vi "CubeDrive.vi"   [LabVIEW 2012]
uses:
  State_Machine_Enum.ctl
  <vilib>/Rock Robotics/WPI/RobotDrive/WPI_RobotDriveGetSetRefNum.vi
  Robot Global Data.vi
types:
  T1 = typedef "State_Machine_Enum.ctl" = enum16{"Idle", "Start", "Do", "Stop", "Init"}
  T2 = typedef "WPI_RobotDriveDevRef.ctl" = cluster{"DevStatus":errorcluster, "Motors[]":T3[], "Square Inputs":bool, "Max Output":dbl, "Isochronous":bool}
  T3 = typedef "WPI_MotorControlDeviceRef.ctl" = cluster{"DeviceStatus":errorcluster, "Type":enum16{"PWM", "CAN"}, "PWM":cluster{"Digital Module":T4, "PWM Channel":T5, "DeadBand":T6}, "CAN":cluster{"Device Number":u8, "Control Mode":T7, "Semaphore":T8, "Max Vout":dbl}, "Invert":bool, "TransformRef":T9, "InvTransformRef":T9}
  T4 = typedef "FPGA_TypedefDigitalModule.ctl" = enum16{"Digital Module 1", "Digital Module 2"}
  T5 = typedef "FPGA_DIOPWMChannel.ctl" = enum8{"PWM 1", "PWM 2", "PWM 3", "PWM 4", "PWM 5", "PWM 6", "PWM 7", "PWM 8", "PWM 9", "PWM 10", "Invalid"}
  T6 = typedef "WPI_PWMDeadband.ctl" = cluster{"Name":string, "maxPositivePwm":i32, "minPositivePwm":i32, "centerPwm":i32, "maxNegativePwm":i32, "minNegativePwm":i32, "angularRange":u16}
  T7 = typedef "WPI_CANJaguar_ControlMode.ctl" = enum8{"Percent VBus", "Current", "Speed", "Position", "Voltage"}
  T8 = typedef "Semaphore RefNum" = refnum<k1>
  T9 = typedef "WPI_PWMTransform_ConPane.ctl" = refnum<vi>
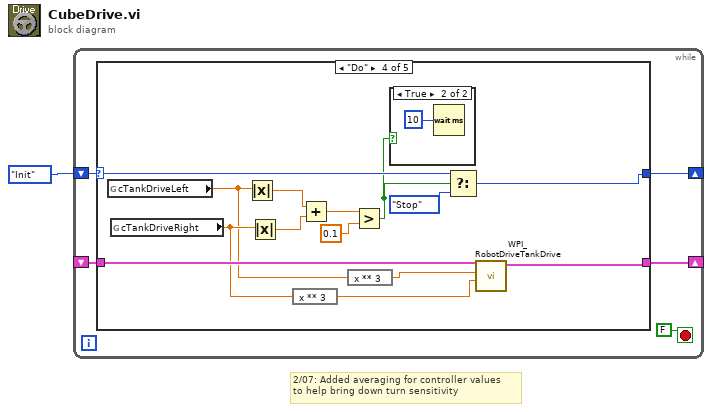
[diagram p0: block diagram]
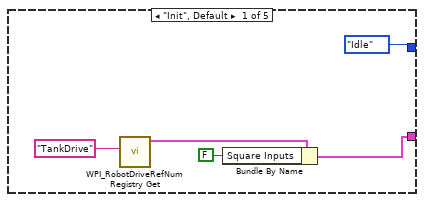
[diagram p2: hidden frame]
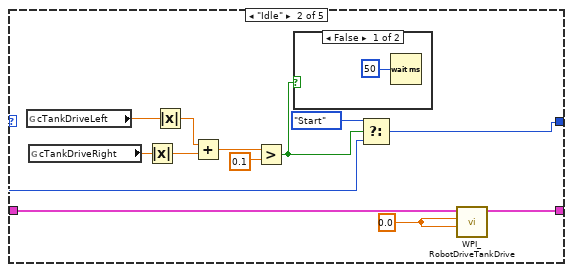
[diagram p3: hidden frame]
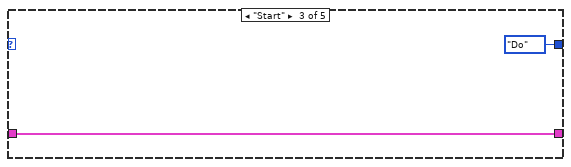
[diagram p5: hidden frame]
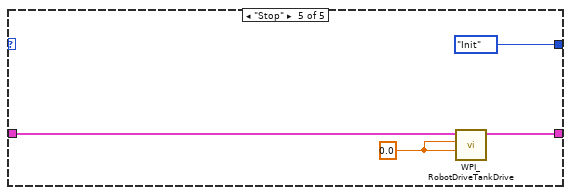
[diagram p7: hidden frame]
diagram:
  # "2/07: Added averaging for controller values\nto help bring down turn sensitivity"
  n1 = while {
    shift-right: [w4] -> _
    shift-left: State_Machine_Enum."Init" ("State") -> [w5]
    shift-right: [w3] -> _
    shift-left: _ -> [w2]
    stop <- FALSE stop-if-true
    n2 = case shown="\"Do\"" w5 {
      selector: w5 -> [_ w17 _ w41 _]
      tunnel: [State_Machine_Enum."Idle" ("State") w16 State_Machine_Enum."Do" ("State") w40 State_Machine_Enum."Init" ("State")] -> w4
      tunnel: [w7 w18 w27 w39 w45] -> w3
      tunnel: w2 -> [_ w19 w27 w32 w44]
      frame "Init", Default {
        n3 = call <vilib>:"WPI_RobotDriveRefNum Registry Get.vi"("refnum name"="TankDrive") -> ("RobotDriveDevRef"=w8:T2)  [unwired: 9 in, 1 out]
        n4 = Bundle By Name(cluster=w8, "Square Inputs"=FALSE) -> (w7:T2)
      }
      frame "Idle" {
        w13 = 0.0 ("Left axis value")
        n5 = global read "Robot Global Data.vi" "cTankDriveLeft"() -> (w15:dbl)
        n6 = global read "Robot Global Data.vi" "cTankDriveRight"() -> (w14:dbl)
        n7 = Absolute Value(x=w14) -> (abs(x)=w23:dbl)
        n8 = Absolute Value(x=w15) -> (abs(x)=w24:dbl)
        n9 = Add(x=w24, y=w23) -> (x+y=w22:dbl)
        n10 = Greater?(x=w22, y=0.1) -> (0:w20:bool)
        n11 = case shown="False" w20 {
          frame False {
            n12 = Wait (ms)(milliseconds to wait=u32 50) -> ()  [unwired: 1 out]
          }
          frame True {
          }
        }
        n13 = Select(t=State_Machine_Enum."Start" ("State"), s=w20, f=w17) -> (s? t:f=w16:T1)
        n14 = call <vilib>:"WPI_RobotDriveTankDrive.vi"("Right axis value"=w13, "Left axis value"=w13, "RobotDriveDevRef"=w19) -> ("RobotDriveDevRef"=w18:T2)  [unwired: 6 in, 2 out]
      }
      frame "Start" {
      }
      frame "Do" {
        n15 = global read "Robot Global Data.vi" "cTankDriveLeft"() -> (w29:dbl)
        n16 = global read "Robot Global Data.vi" "cTankDriveRight"() -> (w31:dbl)
        n17 = Absolute Value(x=w29) -> (abs(x)=w37:dbl)
        n18 = Absolute Value(x=w31) -> (abs(x)=w36:dbl)
        n19 = expression code="x ** 3"(w31) -> (w30:dbl)
        n20 = Add(x=w37, y=w36) -> (x+y=w35:dbl)
        n21 = expression code="x ** 3"(w29) -> (w28:dbl)
        n22 = Greater?(x=w35, y=0.1) -> (0:w33:bool)
        n23 = case shown="True" w33 {
          frame False {
          }
          frame True {
            n24 = Wait (ms)(milliseconds to wait=u32 10) -> ()  [unwired: 1 out]
          }
        }
        n25 = Select(t=w41, s=w33, f=State_Machine_Enum."Stop" ("State")) -> (s? t:f=w40:T1)
        n26 = call <vilib>:"WPI_RobotDriveTankDrive.vi"("Right axis value"=w30, "Left axis value"=w28, "RobotDriveDevRef"=w32) -> ("RobotDriveDevRef"=w39:T2)  [unwired: 6 in, 2 out]
      }
      frame "Stop" {
        w46 = 0.0 ("Left axis value")
        n27 = call <vilib>:"WPI_RobotDriveTankDrive.vi"("Right axis value"=w46, "Left axis value"=w46, "RobotDriveDevRef"=w44) -> ("RobotDriveDevRef"=w45:T2)  [unwired: 6 in, 2 out]
      }
    }
  }
